vi "Launcher.vi"   [LabVIEW 2020]
uses:
  Server/Server/Server.lvclass
  C:/Program Files (x86)/National Instruments/LabVIEW 2020/vi.lib/ActorFramework/Actor/Actor.lvclass
  <vilib>/ActorFramework/Actor/Actor.lvclass
types:
  T1 = enum32{"Invalid", "Standard", "Closed", "Hidden", "Minimized", "Maximized"}
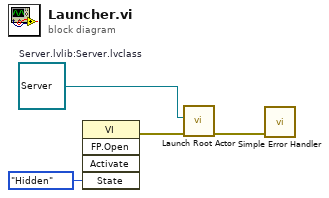
[diagram p0: block diagram]
diagram:
  w4 = refnum<class "Server.lvclass"> refnum  # Server.lvlib:Server.lvclass
  n1 = invoke class="VI" method="FP.Open"("State"=T1."Hidden") -> (error out=w1:errorcluster)  [unwired: 4 in, 4 out]
  n2 = call <vilib>:"Launch Root Actor.vi"("error in (no error)"=w1, "Actor"=w4) -> ("error out"=w3:errorcluster)  [unwired: 8 in, 1 out]
  n3 = call <vilib>:"Simple Error Handler.vi"("error in (no error)"=w3) -> ()  [unwired: 4 in, 5 out]
